vi "TicksPriv.vi"(4 "Tick Properties":T1={"Text"={"Color"=2147483647, "Background Color"=2147483647, "Font Size (points)"=0, "Font Style"=enum."Automatic", "Rotation Angle"=nan}} {"Text"."Background Color" items=["Automatic"=2147483647, "Black"=0, "White"=16777215, "Red"=16711680, "Green"=2263842, "Blue"=255, "Cyan"=65535, "Magenta"=16711935, "Yellow"=16776960]; "Text"."Font Size (points)" items=["Automatic"=0, "XX-Small"=-1, "X-Small"=-2, "Small"=-3, "Medium"=-4, "Large"=-5, "X-Large"=-6, "XX-Large"=-7]; "Text"."Color" items=["Automatic"=2147483647, "Black"=0, "White"=16777215, "Red"=16711680, "Green"=2263842, "Blue"=255, "Cyan"=65535, "Magenta"=16711935, "Yellow"=16776960]}, 7 "Axis":enum16{"X Axis", "Y Axis"}(ring), 8 "error in (no error)":errorcluster, 9 "Tick Labels":string[](array[string]), 10 "Tick Locations":dbl[](array[numeric]), 11 "Plot ID":T6 format="%x") -> (0 "error out":errorcluster)   [LabVIEW 2013, in "Advanced Plotting Toolkit.lvlib"]
uses:
  Advanced Plotting Toolkit.lvlib
  typedefs/PlotID.ctl
  TicksProperties.ctl
  properties/Text.ctl
  typedefs/PlotColor.ctl
  properties/Text_FontSize.ctl
  properties/Text_FontStyle.ctl
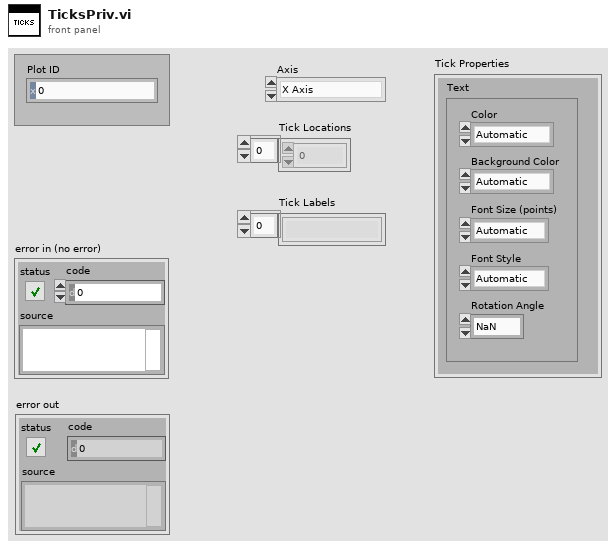
[diagram p1: front panel]
types:
  T1 = typedef "Advanced Plotting Toolkit.lvlib/TicksProperties.ctl" = cluster{"Text":T2}
  T2 = typedef "Advanced Plotting Toolkit.lvlib/Text.ctl" = cluster{"Color":T3, "Background Color":T3, "Font Size (points)":T4, "Font Style":T5, "Rotation Angle":dbl}
  T3 = typedef "Advanced Plotting Toolkit.lvlib/PlotColor.ctl" = u32
  T4 = typedef "Advanced Plotting Toolkit.lvlib/Text_FontSize.ctl" = i32
  T5 = typedef "Advanced Plotting Toolkit.lvlib/Text_FontStyle.ctl" = enum16{"Automatic", "Normal", "Italic", "Bold"}
  T6 = typedef "Advanced Plotting Toolkit.lvlib/PlotID.ctl" = i32
  T7 = typedef "Advanced Plotting Toolkit.lvlib/KeyValue.ctl" = cluster{"Key":string, "Value":string}
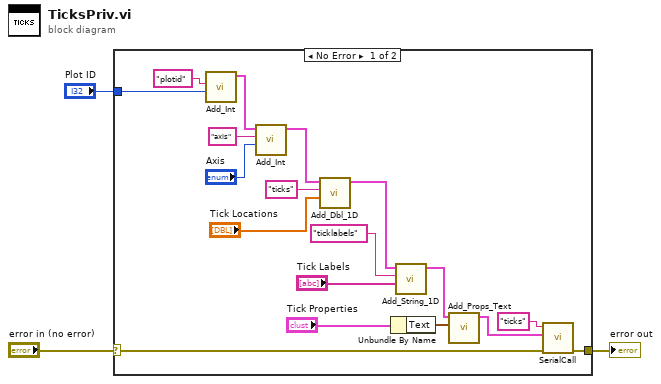
[diagram p0: block diagram]
diagram:
  n1 = case shown="No Error" "error in (no error)" {
    selector: "error in (no error)" -> [w11 w22]
    tunnel: "Plot ID" -> [w14 _]
    tunnel: [w10 w22] -> w1
    frame No Error {
      n2 = call "Add_Int.vi"("Value"=w14, "Key"="plotid") -> ("Keyword Array Out"=w9:T7[])  [unwired: 9 in]
      n3 = call "Add_Int.vi"("Value"="Axis", "Key"="axis", "Keyword Array"=w9) -> ("Keyword Array Out"=w8:T7[])  [unwired: 8 in]
      n4 = call "Add_Dbl_1D.vi"("Value"="Tick Locations", "Key"="ticks", "Keyword Array"=w8) -> ("Keyword Array Out"=w17:T7[])  [unwired: 8 in]
      n5 = Unbundle By Name("Tick Properties") -> ("Text"=w4:T2)
      n6 = call "Add_String_1D.vi"("Value"="Tick Labels", "Key"="ticklabels", "Keyword Array"=w17) -> ("Keyword Array Out"=w16:T7[])  [unwired: 8 in]
      n7 = call "Add_Props_Text.vi"("Text Properties"=w4, "Keyword Array"=w16) -> ("Keyword Array Out"=w13:T7[])  [unwired: 9 in]
      n8 = call "SerialCall.vi"("error in (no error)"=w11, "data"=w13, "Resource"="ticks") -> ("error out"=w10:errorcluster)  [unwired: 7 in, 1 out]
    }
    frame Error {
    }
  }
  "error out" <- w1
